vi "16-ParsePacket.vi"(11 "BITS in":bool[](array[boolean])) -> (2 "Packet":T1, 3 "BITS out":bool[](array[boolean]))   [LabVIEW 2019, in "16.lvlib"]
uses:
  16.lvlib
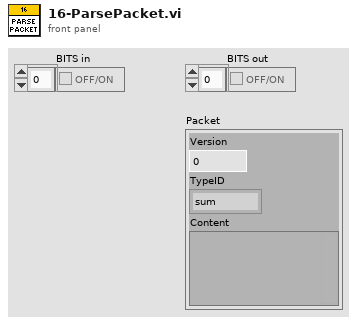
[diagram p1: front panel]
types:
  T1 = cluster{"Version":u32, "TypeID":enum16{"sum", "product", "minimum", "maximum", "literal", "greater than", "less than", "equal to"}, "Content":variant}
  T2 = enum16{"sum", "product", "minimum", "maximum", "literal", "greater than", "less than", "equal to"}
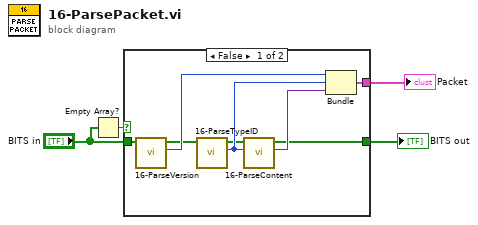
[diagram p0: block diagram]
diagram:
  n1 = Empty Array?(array="BITS in") -> (empty?=w1:bool)
  n2 = case shown="False" w1 {
    tunnel: [w10 w13] -> w4
    tunnel: [w8 _] -> w3
    tunnel: "BITS in" -> [w5 w13]
    frame False {
      n3 = call "16-ParseVersion.vi"("BITS in"=w5) -> ("Version"=w7:u32, "BITS out"=w6:bool[])  [unwired: 9 in]
      n4 = call "16-ParseTypeID.vi"("BITS in"=w6) -> ("TypeID"=w11:T2, "BITS out"=w9:bool[])  [unwired: 9 in]
      n5 = call "16-ParseContent.vi"("TypeID"=w11, "BITS in"=w9) -> ("Content"=w12:variant, "BITS out"=w10:bool[])  [unwired: 8 in]
      n6 = Bundle("Version"=w7, "TypeID"=w11, "Content"=w12) -> (w8:T1)  [unwired: 1 in]
    }
    frame True {
    }
  }
  "BITS out" <- w4
  "Packet" <- w3
